vi "GetRunStopTime.vi"(0 "Timeout after n trys (default = 100 (10s))":i32=100, 1 "error in (no error)":errorcluster) -> (2 "Run Stop Time (UNIX Time)":u32, 3 "Run Stop Time":timestamp, 4 "error out":errorcluster)   [LabVIEW 2018]
uses:
  DataPacker/Utilities/PeriodicEnumTypeDef.ctl
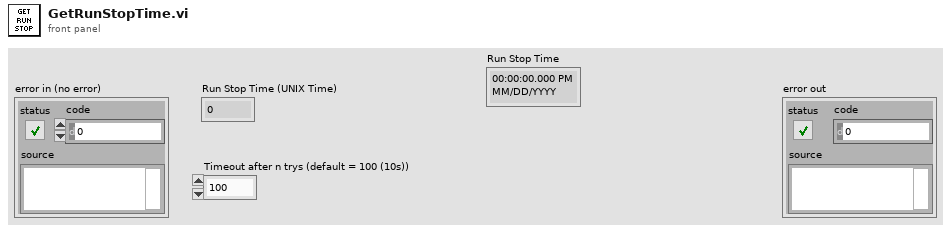
[diagram p1: front panel]
types:
  T1 = typedef "PeriodicEnumTypeDef.ctl" = enum16{"GET_STATUS", "GET_HIST_RATE", "GET_RUNNO", "GET_RUN_START_T", "GET_RUN_STOP_T", "GET_TIME"}
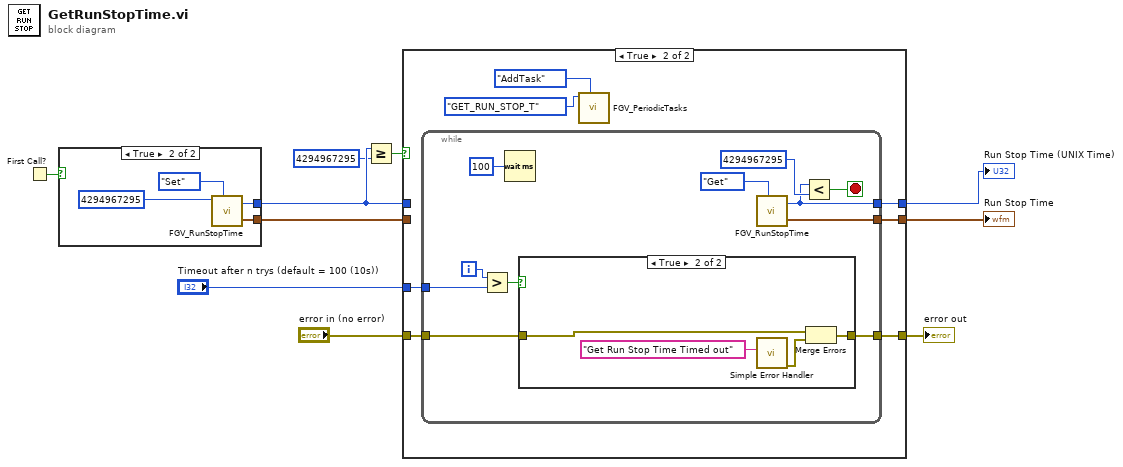
[diagram p0: block diagram]
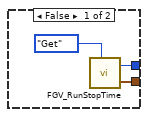
[diagram p2: hidden frame]
diagram:
  n1 = First Call?() -> (First Call?: T/F=w6:bool)
  n2 = case shown="True" w6 {
    tunnel: [w13 w15] -> w5
    tunnel: [w12 w14] -> w1
    frame False {
      n3 = call "FGV_RunStopTime.vi"("Enum"=enum16{"Set", "Get"}."Get") -> ("Run Stop Time (UNIX Time)"=w13:u32, "Run Stop Time (UTC)"=w12:timestamp)  [unwired: 4 in]
    }
    frame True {
      n4 = call "FGV_RunStopTime.vi"("Run Stop Time"=u32 4294967295 ("Run Start Time"), "Enum"=enum16{"Set", "Get"}."Set") -> ("Run Stop Time (UNIX Time)"=w15:u32, "Run Stop Time (UTC)"=w14:timestamp)  [unwired: 3 in]
    }
  }
  n5 = Greater Or Equal?(x=w5, y=u32 4294967295) -> (x >= y?=w4:bool)
  n6 = case shown="True" w4 {
    tunnel: [w20 w27] -> w10
    tunnel: w5 -> [w20 _]
    tunnel: "error in (no error)" -> [w19 w26]
    tunnel: [w19 w25] -> w9
    tunnel: "Timeout after n trys (default = 100 (10s))" -> [_ w22]
    tunnel: [w18 w21] -> w2
    tunnel: w1 -> [w18 _]
    frame False {
    }
    frame True {
      n7 = while {
        tunnel: [w29] -> w27
        tunnel: w26 -> [w35]
        tunnel: [w34] -> w25
        tunnel: w22 -> [w33]
        tunnel: [w30] -> w21
        i -> [w37]
        stop <- w31 stop-if-true
        n8 = Greater?(x=w37, y=w33) -> (0:w36:bool)
        n9 = Wait (ms)(milliseconds to wait=u32 100) -> ()  [unwired: 1 out]
        n10 = case shown="True" w36 {
          tunnel: w35 -> [w39 w42]
          tunnel: [w39 w40] -> w34
          frame False {
          }
          frame True {
            n11 = call <vilib>:"Simple Error Handler.vi"("error source (\" \")"="Get Run Stop Time Timed out" ("error source (\" \")")) -> ("error out"=w41:errorcluster)  [unwired: 4 in, 4 out]
            n12 = Merge Errors(w42, w41) -> (w40:errorcluster)
          }
        }
        n13 = call "FGV_RunStopTime.vi"("Enum"=enum16{"Set", "Get"}."Get") -> ("Run Stop Time (UNIX Time)"=w29:u32, "Run Stop Time (UTC)"=w30:timestamp)  [unwired: 4 in]
        n14 = Less?(x=w29, y=u32 4294967295) -> (x < y?=w31:bool)
      }
      n15 = call "FGV_PeriodicTasks.vi"("MIDAS Commands"=PeriodicEnumTypeDef."GET_RUN_STOP_T" ("Enum"), "Task"=enum16{"AddTask", "GetTasks", "ClearTasks"}."AddTask" ("Enum 2")) -> ()  [unwired: 3 in, 1 out]
    }
  }
  "error out" <- w9
  "Run Stop Time (UNIX Time)" <- w10
  "Run Stop Time" <- w2
